vi "RelayControl_Port_Control.vi"(10 "打开/关闭":enum16{"打开", "关闭"}(ring), 11 "端口号":refnum<visa-resource-name> caption="VISA资源名称") -> ()   [LabVIEW 2013]
uses:
  <vilib>/Instr/_visa.llb/VISA Configure Serial Port (Instr).vi
panel:
  out "error out":errorcluster caption="错误输出"
  in  "error in (no error)":errorcluster caption="错误输入（无错误）"
  out "连接状态":bool
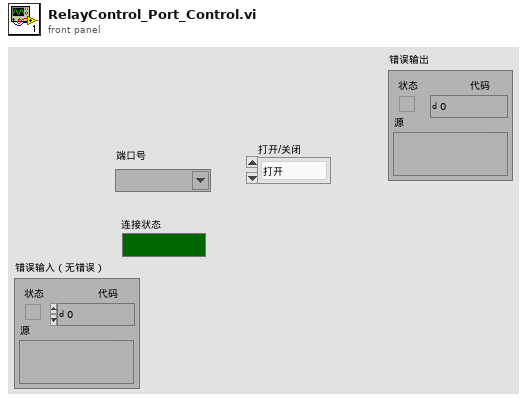
[diagram p1: front panel]
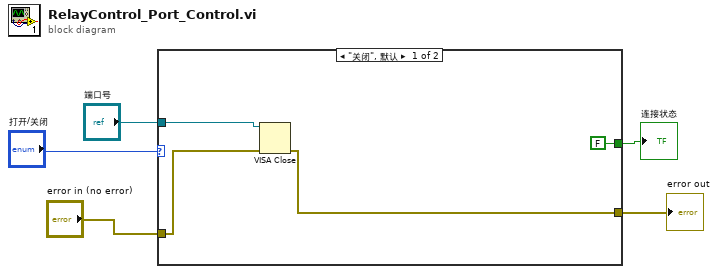
[diagram p0: block diagram]
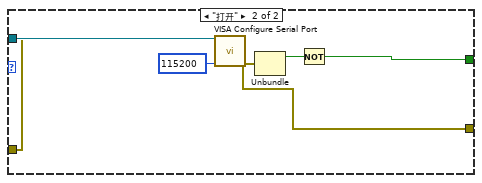
[diagram p2: hidden frame]
diagram:
  n1 = case shown="\"关闭\", 默认" "打开/关闭" {
    tunnel: "端口号" -> [w9 w13]
    tunnel: [FALSE w12] -> w4
    tunnel: "error in (no error)" -> [w6 w11]
    tunnel: [w7 w10] -> w1
    frame "关闭", Default {
      n2 = VISA Close(VISA resource name=w9, error in (no error)=w6) -> (error out=w7:errorcluster)
    }
    frame "打开" {
      n3 = call-poly "VISA Configure Serial Port"("VISA resource name"=w13, "baud rate (9600)"=u32 115200, "error in (no error)"=w11) -> ("error out"=w10:errorcluster)  [unwired: 11 in, 1 out]
      n4 = Unbundle(w10) -> ("status"=w14:bool)  [unwired: 2 out]
      n5 = Not(x=w14) -> (.not. x?=w12:bool)
    }
  }
  "连接状态" <- w4
  "error out" <- w1
